vi "uSec.vi"(2 "error in (no error)":errorcluster) -> (20 "Tick Count(uSec)":u32, 22 "error out":errorcluster)   [LabVIEW 2011]
doc: "Returns uSec tick count.\n\n\nVersion 1.0 - 02/13/2013\n\nPhaeron, Inc.\nwww.phaeron.com\ninfo@phaeron.com"
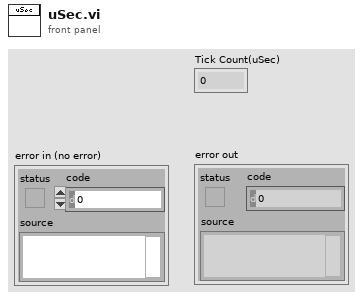
[diagram p1: front panel]
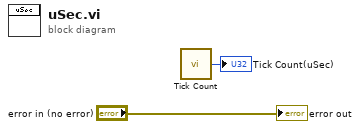
[diagram p0: block diagram]
diagram:
  n1 = call "Tick Count"() -> ("Tick Count(uSec)"=→"Tick Count(uSec)":u32)
  "error out" <- "error in (no error)"
